vi "New Save.vi"() -> ()   [LabVIEW 2017]
panel:
  out "Waveform Graph 2":dbl[](graph)
  in  "Path 2":path
  out "Waveform Graph":dynamicdata(graph)
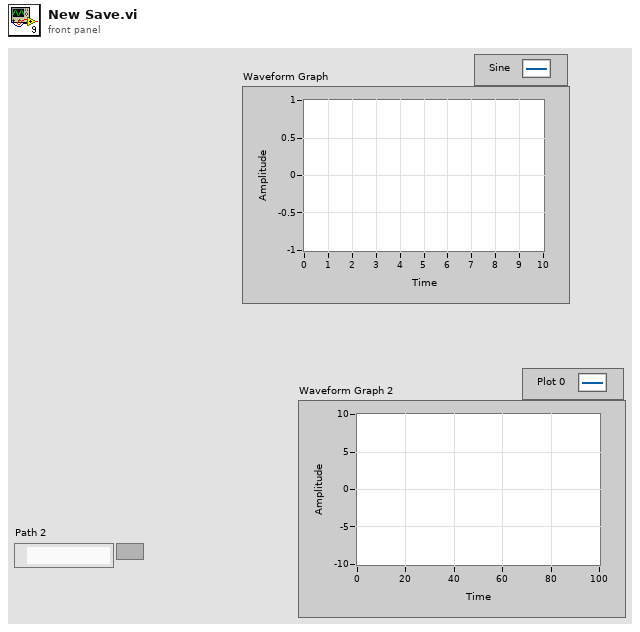
[diagram p1: front panel]
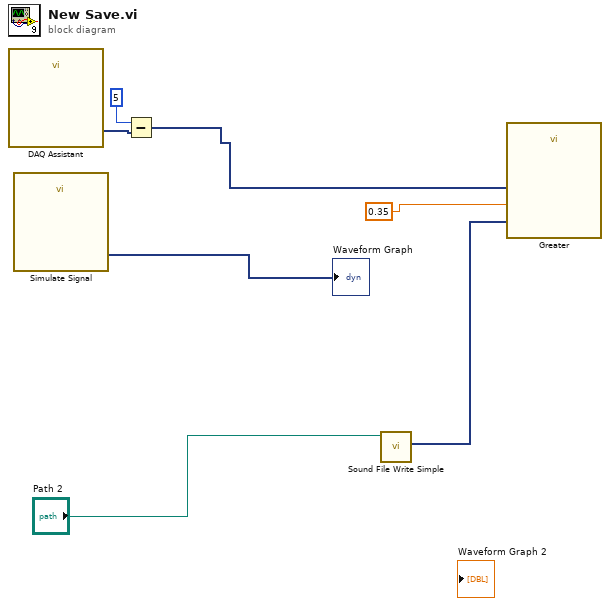
[diagram p0: block diagram]
diagram:
  n1 = call "DAQ Assistant"() -> ("data"=w5:dynamicdata)  [unwired: 17 in, 2 out]
  n2 = call "Simulate Signal"() -> ("Sine"=→"Waveform Graph":dynamicdata)  [unwired: 14 in, 1 out]
  n3 = Subtract(x=5, y=w5) -> (x-y=w3:dynamicdata)
  n4 = call "Greater"("Constant Value to Compare Against"=0.35, "Operand 1"=w3) -> ("Result"=w1:dynamicdata)  [unwired: 8 in, 1 out]
  n5 = call <vilib>:"Sound File Write Simple.vi"("data"=w1, "path"="Path 2") -> ()  [unwired: 8 in, 2 out]
